vi "Lab Panel V5.28.vi"() -> ()   [LabVIEW 2013] (continued)
              n182 = local write "LAB deg C"(w197) -> ()
              n183 = global write "Global display 4.vi" "LAB deg C"(w197) -> ()
              n184 = local write "OFF amps"(1.5) -> ()
              n185 = local write "ON amps"(20.0) -> ()
              n186 = local write "VOLTS"(250.0) -> ()
              n187 = local write "PF"(0.5) -> ()
            }
            frame #1 {
              n188 = for {
                N: 3 -> [_]
                w243 = TRUE
                n189 = local read "Simulate"() -> (w205:bool)
                n190 = local write "Temp read loop"(0) -> ()
                n191 = case shown="True" w205 {
                  frame False {
                  }
                  frame True {
                    w245 = 20
                    n192 = local write "Ambient Volts"(2.92) -> ()
                    n193 = global write "Global display 3.vi" "Ref deg C"(w245) -> ()
                    n194 = local write "Ref deg C"(w245) -> ()
                  }
                }
                n195 = call "sub vi - GET ALL TEMP v7.vi"("LA01-EN"=w243, "simulate"=w205, "LA02-EN"=w243, "LA03-EN"=w243, "LA04-EN"=w243, "LA05-EN"=w243, "Gen Cal Value"=1) -> ("ID"=w204:T24, "LA01 TEMP"=w241:T25, "LA02 TEMP"=w234:T25, "LA03 TEMP"=w227:T25, "LA04 TEMP"=w220:T25, "LA05 TEMP"=w213:T25)  [unwired: 1 in, 2 out]
                n196 = local write "LAB05 TEMP"(w213) -> ()
                n197 = local write "LAB04 TEMP"(w220) -> ()
                n198 = Unbundle(w227) -> ("T1"=w224:dbl, "T2"=w223:dbl, "T3"=w222:dbl, "T4"=w221:dbl)  [unwired: 2 out]
                n199 = Unbundle(w241) -> ("T1"=w239:dbl, "T2"=w238:dbl, "T3"=w237:dbl, "T4"=w236:dbl)  [unwired: 2 out]
                n200 = Unbundle(w234) -> ("T1"=w231:dbl, "T2"=w230:dbl, "T3"=w229:dbl, "T4"=w228:dbl)  [unwired: 2 out]
                n201 = Unbundle(w220) -> ("T1"=w218:dbl, "T2"=w217:dbl, "T3"=w216:dbl, "T4"=w215:dbl)  [unwired: 2 out]
                n202 = Unbundle(w213) -> ("T1"=w211:dbl, "T2"=w210:dbl, "T3"=w209:dbl, "T4"=w208:dbl)  [unwired: 2 out]
                n203 = local write "LAB01 TEMP"(w241) -> ()
                n204 = local write "LAB02 TEMP"(w234) -> ()
                n205 = local write "LAB03 TEMP"(w227) -> ()
                n206 = Unbundle(w204) -> ("id1"=→"LAB01-TP":bool, "id2"=→"LAB02-TP":bool, "id3"=→"LAB03-TP":bool, "id4"=→"LAB04-TP":bool, "id5"=→"LAB05-TP":bool)
                n207 = local read "TEMP LA05"() -> (w212:T9)
                n208 = local read "TEMP LA04"() -> (w219:T9)
                n209 = local read "TEMP LA02"() -> (w233:T9)
                n210 = local read "TEMP LA03"() -> (w226:T9)
                n211 = local read "TEMP LA01"() -> (w240:T9)
                n212 = Bundle(cluster=w226, "TL-1"=w224, "TN-1"=w223, "TL-2"=w222, "TN-2"=w221) -> (w225:T9)  [unwired: 4 in]
                n213 = Bundle(cluster=w240, "TL-1"=w239, "TN-1"=w238, "TL-2"=w237, "TN-2"=w236) -> (w235:T9)  [unwired: 4 in]
                n214 = Bundle(cluster=w233, "TL-1"=w231, "TN-1"=w230, "TL-2"=w229, "TN-2"=w228) -> (w232:T9)  [unwired: 4 in]
                n215 = Bundle(cluster=w219, "TL-1"=w218, "TN-1"=w217, "TL-2"=w216, "TN-2"=w215) -> (w214:T9)  [unwired: 4 in]
                n216 = Bundle(cluster=w212, "TL-1"=w211, "TN-1"=w210, "TL-2"=w209, "TN-2"=w208) -> (w207:T9)  [unwired: 4 in]
                n217 = local write "TEMP LA03"(w225) -> ()
                n218 = local write "TEMP LA01"(w235) -> ()
                n219 = local write "TEMP LA02"(w232) -> ()
                n220 = local write "TEMP LA05"(w207) -> ()
                n221 = local write "TEMP LA04"(w214) -> ()
              }
            }
            frame #2 {
              w254 = 0
              n222 = local read "LAB01 TEMP"() -> (w256:T12)
              n223 = local read "SIG LAB01-2"() -> (w251:T2)
              n224 = Unbundle By Name(w256) -> ("T1 Live"=w249:dbl, "T1 Neut"=w248:dbl, "T2 Live"=w247:dbl, "T2 Neut"=w246:dbl)  [unwired: 2 out]
              n225 = local read "SIG LAB01-1"() -> (w253:T2)
              n226 = local read "TEMP LA01"() -> (w257:T9)
              n227 = Bundle By Name(cluster=w257, "TL-1"=w249, "TN-1"=w248, "TL-2"=w247, "TN-2"=w246, "TL -1COUNT"=w254, "TN-1 COUNT"=w254, "TL-2 COUNT"=w254, "TN-2 COUNT"=w254) -> (w255:T9)
              n228 = Bundle(cluster=w253, "Tmp Live"=w249, "Tmp Neut"=w248) -> (w252:T2)  [unwired: 3 in]
              n229 = Bundle(cluster=w251, "Tmp Live"=w247, "Tmp Neut"=w246) -> (w250:T2)  [unwired: 3 in]
              n230 = local write "SIG LAB01-2"(w250) -> ()
              n231 = local write "SIG LAB01-1"(w252) -> ()
              n232 = local write "TEMP LA01"(w255) -> ()
            }
            frame #3 {
              w266 = 0
              n233 = local read "LAB02 TEMP"() -> (w268:T12)
              n234 = Unbundle By Name(w268) -> ("T1 Live"=w261:dbl, "T1 Neut"=w260:dbl, "T2 Live"=w259:dbl, "T2 Neut"=w258:dbl)  [unwired: 2 out]
              n235 = local read "SIG LAB02-1"() -> (w265:T2)
              n236 = local read "SIG LAB02-2"() -> (w264:T2)
              n237 = local read "TEMP LA02"() -> (w269:T9)
              n238 = Bundle By Name(cluster=w269, "TL-1"=w261, "TN-1"=w260, "TL-2"=w259, "TN-2"=w258, "TL -1COUNT"=w266, "TN-1 COUNT"=w266, "TL-2 COUNT"=w266, "TN-2 COUNT"=w266) -> (w267:T9)
              n239 = Bundle(cluster=w264, "Tmp Live"=w259, "Tmp Neut"=w258) -> (w262:T2)  [unwired: 3 in]
              n240 = Bundle(cluster=w265, "Tmp Live"=w261, "Tmp Neut"=w260) -> (w263:T2)  [unwired: 3 in]
              n241 = local write "TEMP LA02"(w267) -> ()
              n242 = local write "SIG LAB02-1"(w263) -> ()
              n243 = local write "SIG LAB02-2"(w262) -> ()
            }
            frame #4 {
              w278 = 0
              n244 = local read "LAB03 TEMP"() -> (w280:T12)
              n245 = Unbundle By Name(w280) -> ("T1 Live"=w273:dbl, "T1 Neut"=w272:dbl, "T2 Live"=w271:dbl, "T2 Neut"=w270:dbl)  [unwired: 2 out]
              n246 = local read "SIG LAB03-1"() -> (w277:T2)
              n247 = local read "SIG LAB03-2"() -> (w276:T2)
              n248 = local read "TEMP LA03"() -> (w281:T9)
              n249 = Bundle By Name(cluster=w281, "TL-1"=w273, "TN-1"=w272, "TL-2"=w271, "TN-2"=w270, "TL -1COUNT"=w278, "TN-1 COUNT"=w278, "TL-2 COUNT"=w278, "TN-2 COUNT"=w278) -> (w279:T9)
              n250 = Bundle(cluster=w276, "Tmp Live"=w271, "Tmp Neut"=w270) -> (w274:T2)  [unwired: 3 in]
              n251 = Bundle(cluster=w277, "Tmp Live"=w273, "Tmp Neut"=w272) -> (w275:T2)  [unwired: 3 in]
              n252 = local write "TEMP LA03"(w279) -> ()
              n253 = local write "SIG LAB03-2"(w274) -> ()
              n254 = local write "SIG LAB03-1"(w275) -> ()
            }
            frame #5 {
              w290 = 0
              n255 = local read "LAB04 TEMP"() -> (w292:T12)
              n256 = Unbundle By Name(w292) -> ("T1 Live"=w285:dbl, "T1 Neut"=w284:dbl, "T2 Live"=w283:dbl, "T2 Neut"=w282:dbl)  [unwired: 2 out]
              n257 = local read "SIG LAB04-2"() -> (w288:T2)
              n258 = local read "SIG LAB04-1"() -> (w289:T2)
              n259 = local read "TEMP LA04"() -> (w293:T9)
              n260 = Bundle By Name(cluster=w293, "TL-1"=w285, "TN-1"=w284, "TL-2"=w283, "TN-2"=w282, "TL -1COUNT"=w290, "TN-1 COUNT"=w290, "TL-2 COUNT"=w290, "TN-2 COUNT"=w290) -> (w291:T9)
              n261 = Bundle(cluster=w288, "Tmp Live"=w283, "Tmp Neut"=w282) -> (w286:T2)  [unwired: 3 in]
              n262 = Bundle(cluster=w289, "Tmp Live"=w285, "Tmp Neut"=w284) -> (w287:T2)  [unwired: 3 in]
              n263 = local write "SIG LAB04-2"(w286) -> ()
              n264 = local write "TEMP LA04"(w291) -> ()
              n265 = local write "SIG LAB04-1"(w287) -> ()
            }
            frame #6 {
              w302 = 0
              n266 = local read "LAB05 TEMP"() -> (w304:T12)
              n267 = Unbundle By Name(w304) -> ("T1 Live"=w297:dbl, "T1 Neut"=w296:dbl, "T2 Live"=w295:dbl, "T2 Neut"=w294:dbl)  [unwired: 2 out]
              n268 = local read "SIG LAB05-2"() -> (w300:T2)
              n269 = local read "SIG LAB05-1"() -> (w301:T2)
              n270 = local read "TEMP LA05"() -> (w305:T9)
              n271 = Bundle By Name(cluster=w305, "TL-1"=w297, "TN-1"=w296, "TL-2"=w295, "TN-2"=w294, "TL -1COUNT"=w302, "TN-1 COUNT"=w302, "TL-2 COUNT"=w302, "TN-2 COUNT"=w302) -> (w303:T9)
              n272 = Bundle(cluster=w300, "Tmp Live"=w295, "Tmp Neut"=w294) -> (w298:T2)  [unwired: 3 in]
              n273 = Bundle(cluster=w301, "Tmp Live"=w297, "Tmp Neut"=w296) -> (w299:T2)  [unwired: 3 in]
              n274 = local write "SIG LAB05-2"(w298) -> ()
              n275 = local write "SIG LAB05-1"(w299) -> ()
              n276 = local write "TEMP LA05"(w303) -> ()
            }
          }
        }
        frame #11 {
          # "create analog task"
          n277 = local read "Simulate"() -> (w306:bool)
          n278 = case shown="False" w306 {
            frame False {
              n279 = local read "SAMPLES"() -> (w309:dbl)
              n280 = local read "RATE (Hz)"() -> (w310:dbl)
              n281 = call "sub vi - AI USB4704 (3)  Create Task v4.vi"("Rate Hz"=w310, "Samples"=w309) -> ("TASK USB 0"=→"AI Task0":i32, "TASK USB 1"=→"AI Task1":i32, "TASK USB 2"=→"AI Task2":i32, "AI Task Er"=w307:bool)  [unwired: 9 in, 1 out]
              n282 = local write "Reset Error"(w307) -> ()
              "AI Task" <- TRUE
            }
            frame True {
            }
          }
        }
        frame #12 {
          # "enable front panel, all settings done"
          n283 = property on="Tab Control 2" class="TabCtl (strict)"("DisabledEnum"=T16."Enabled" ("Disabled")) -> ()  [unwired: 2 in, 2 out]
          n284 = property on="Tab Control 2" class="TabCtl (strict)"("Value"=0) -> ()  [unwired: 2 in, 2 out]
        }
        frame #13 {
          n285 = property on="Tab Control 2" class="TabCtl (strict)"("Value"=0) -> ()  [unwired: 2 in, 2 out]
        }
      }
    }
    frame #2 {
      w317 = 250.0
      # "frames that only action on certain cycles, 13, 14, 15, 16, 19, 21"
      n286 = node-c288(w317) -> (w319:T18)  [unwired: 3 in]
      n287 = timed-loop {
        timing: w319 -> [_]
        timing-out: [_] -> w318
        tunnel: w317 -> [w320]
        i -> [w346]
        stop <- w321 stop-if-true
        n288 = node-c288() -> ()  [unwired: 1 in, 1 out]
        n289 = local read "Resets Done"() -> (w325:dbl)
        n290 = local read "SELECT LAB05-2"() -> (w326:T3)
        n291 = local read "SELECT LAB05-1"() -> (w327:T3)
        n292 = local read "SELECT LAB04-2"() -> (w328:T3)
        n293 = local read "SELECT LAB03-1"() -> (w331:T3)
        n294 = local read "SELECT LAB02-2"() -> (w332:T3)
        n295 = local read "SELECT LAB01-1"() -> (w335:T3)
        n296 = local read "SELECT LAB03-2"() -> (w330:T3)
        n297 = local read "SELECT LAB01-2"() -> (w334:T3)
        n298 = local read "SELECT LAB04-1"() -> (w329:T3)
        n299 = Greater?(x=w325, y=50) -> (0:w322:bool)
        n300 = local read "SELECT LAB02-1"() -> (w333:T3)
        n301 = local read "run lab03-2"() -> (w340:bool)
        n302 = local read "run lab04-1"() -> (w339:bool)
        n303 = local read "run lab05-1"() -> (w337:bool)
        n304 = local read "run lab04-2"() -> (w338:bool)
        n305 = local read "run lab05-2"() -> (w336:bool)
        n306 = local read "run lab03-1"() -> (w341:bool)
        n307 = local read "run lab02-2"() -> (w342:bool)
        n308 = local read "run lab02-1"() -> (w343:bool)
        n309 = local read "run lab01-1"() -> (w345:bool)
        n310 = local read "run lab01-2"() -> (w344:bool)
        n311 = Or(x=w322, y="stop") -> (x .or. y?=w321:bool)
        n312 = global write "Global display 1.vi" "stop disp"(w321) -> ()
        n313 = stacked-sequence {
          seq-local: [_ _ w425 _ _ _ _ _ _ _ _ _ _ _ _ _ _ _ _ _ _ _ _ _ _] -> [_ _ _ _ _ _ w2526 _ _ _ _ _ _ _ _ _ _ _ _ _ _ _ _ _ _]
          seq-local: [_ _ w424 _ _ _ _ _ _ _ _ _ _ _ _ _ _ _ _ _ _ _ _ _ _] -> [_ _ _ _ _ _ w2525 _ _ _ _ _ _ _ _ _ _ _ _ _ _ _ _ _ _]
          seq-local: [_ _ w411 _ _ _ _ _ _ _ _ _ _ _ _ _ _ _ _ _ _ _ _ _ _] -> [_ _ _ _ _ _ w2524 _ _ _ _ _ _ _ _ _ _ _ _ _ _ _ _ _ _]
          seq-local: [_ _ w410 _ _ _ _ _ _ _ _ _ _ _ _ _ _ _ _ _ _ _ _ _ _] -> [_ _ _ _ _ _ w2523 _ _ _ _ _ _ _ _ _ _ _ _ _ _ _ _ _ _]
          seq-local: [_ _ w409 _ _ _ _ _ _ _ _ _ _ _ _ _ _ _ _ _ _ _ _ _ _] -> [_ _ _ _ _ _ w2522 _ _ _ _ _ _ _ _ _ _ _ _ _ _ _ _ _ _]
          seq-local: [_ _ w408 _ _ _ _ _ _ _ _ _ _ _ _ _ _ _ _ _ _ _ _ _ _] -> [_ _ _ _ _ _ w2521 _ _ _ _ _ _ _ _ _ _ _ _ _ _ _ _ _ _]
          seq-local: [_ _ w407 _ _ _ _ _ _ _ _ _ _ _ _ _ _ _ _ _ _ _ _ _ _] -> [_ _ _ _ _ _ w2520 _ _ _ _ _ _ _ _ _ _ _ _ _ _ _ _ _ _]
          seq-local: [_ _ w406 _ _ _ _ _ _ _ _ _ _ _ _ _ _ _ _ _ _ _ _ _ _] -> [_ _ _ _ _ _ w2519 _ _ _ _ _ _ _ _ _ _ _ _ _ _ _ _ _ _]
          seq-local: [_ _ w405 _ _ _ _ _ _ _ _ _ _ _ _ _ _ _ _ _ _ _ _ _ _] -> [_ _ _ _ _ _ w2518 _ _ _ _ _ _ _ _ _ _ _ _ _ _ _ _ _ _]
          seq-local: [_ _ w404 _ _ _ _ _ _ _ _ _ _ _ _ _ _ _ _ _ _ _ _ _ _] -> [_ _ _ _ _ _ w2517 _ _ _ _ _ _ _ _ _ _ _ _ _ _ _ _ _ _]
          seq-local: [_ _ _ _ _ _ _ _ _ _ _ _ w3660 _ _ _ _ _ _ _ _ _ _ _ _] -> [_ _ _ _ _ _ _ _ _ _ _ _ _ w3692 _ _ _ _ _ _ _ _ _ _ _]
          tunnel: w345 -> [_ _ _ w441 w689 w2116 w2546 w2862 w3349 _ _ _ _ _ w3976 _ w4933 _ _ w5224 w5528 w5709 _ _ _]
          tunnel: w344 -> [_ _ _ w440 w687 w2115 w2545 w2863 w3348 _ _ _ _ _ w3975 _ w4931 _ _ w5223 w5527 w5707 _ _ _]
          tunnel: w343 -> [_ _ _ w439 w685 w2114 w2544 w2861 w3347 _ _ _ _ _ w3974 _ w4929 _ _ w5222 w5526 w5706 _ _ _]
          tunnel: w342 -> [_ _ _ w438 w683 w2113 w2543 w2860 w3346 _ _ _ _ _ w3973 _ w4927 _ _ w5221 w5525 w5705 _ _ _]
          tunnel: w341 -> [_ _ _ w437 w681 w2112 w2542 w2859 w3345 _ _ _ _ _ w3972 _ w4925 _ _ w5220 w5524 w5704 _ _ _]
          tunnel: w340 -> [_ _ _ w436 w679 w2111 w2541 w2858 w3344 _ _ _ _ _ w3971 _ w4923 _ _ w5219 w5523 w5703 _ _ _]
          tunnel: w339 -> [_ _ _ w435 w677 w2110 w2540 w2857 w3343 _ _ _ _ _ w3970 _ w4921 _ _ w5218 w5522 w5702 _ _ _]
          tunnel: w338 -> [_ _ _ w434 w675 w2109 w2539 w2856 w3342 _ _ _ _ _ w3969 _ w4919 _ _ w5217 w5521 w5701 _ _ _]
          tunnel: w337 -> [_ _ _ w433 w673 w2108 w2538 w2855 w3341 _ _ _ _ _ w3968 _ w4917 _ _ w5216 w5520 w5700 _ _ _]
          tunnel: w336 -> [_ _ _ w432 w671 w2107 w2537 w2854 w3340 _ _ _ _ _ w3967 _ w4915 _ _ w5215 w5519 w5699 _ _ _]
          tunnel: w335 -> [_ _ _ _ w688 w2106 w2536 _ _ _ _ _ _ _ _ _ w4935 _ _ _ _ _ w6165 _ _]
          tunnel: w334 -> [_ _ _ _ w686 w2105 w2535 _ _ _ _ _ _ _ _ _ w4930 _ _ _ _ _ w6164 _ _]
          tunnel: w333 -> [_ _ _ _ w684 w2104 w2534 _ _ _ _ _ _ _ _ _ w4928 _ _ _ _ _ w6163 _ _]
          tunnel: w332 -> [_ _ _ _ w682 w2103 w2533 _ _ _ _ _ _ _ _ _ w4926 _ _ _ _ _ w6162 _ _]
          tunnel: w331 -> [_ _ _ _ w680 w2102 w2532 _ _ _ _ _ _ _ _ _ w4924 _ _ _ _ _ w6161 _ _]
          tunnel: w330 -> [_ _ _ _ w678 w2101 w2531 _ _ _ _ _ _ _ _ _ w4922 _ _ _ _ _ w6160 _ _]
          tunnel: w329 -> [_ _ _ _ w676 w2100 w2530 _ _ _ _ _ _ _ _ _ w4920 _ _ _ _ _ w6159 _ _]
          tunnel: w328 -> [_ _ _ _ w674 w2099 w2529 _ _ _ _ _ _ _ _ _ w4918 _ _ _ _ _ w6158 _ _]
          tunnel: w327 -> [_ _ _ _ w672 w2098 w2528 _ _ _ _ _ _ _ _ _ w4916 _ _ _ _ _ w6157 _ _]
          tunnel: w326 -> [_ _ _ _ w670 w2097 w2527 _ _ _ _ _ _ _ _ _ w4914 _ _ _ _ _ w6156 _ _]
          tunnel: w322 -> [_ _ _ _ _ _ _ _ _ _ _ _ _ _ _ _ _ _ _ _ _ _ _ _ w6268]
          tunnel: w321 -> [_ _ _ _ _ _ _ _ _ _ _ _ _ _ _ _ _ _ _ _ _ _ _ _ w6267]
          tunnel: w320 -> [_ w361 _ _ _ _ _ _ _ _ _ _ _ _ _ _ _ _ _ _ _ _ _ _ _]
          frame #0 {
            n314 = local read "AI Task"() -> (w349:bool)
            n315 = global write "Global 1.vi" "RATE(Hz)"("RATE (Hz)") -> ()
            n316 = case shown="True" w349 {
              frame False {
              }
              frame True {
                n317 = local read "SAMPLES"() -> (w351:dbl)
                n318 = local read "AI Task2"() -> (w357:dbl)
                n319 = local read "AI Task1"() -> (w358:dbl)
                n320 = local read "AI Task0"() -> (w359:dbl)
                n321 = call "sub vi - AI USB4704 (3) v73.vi"("Task0"=w359, "Task1"=w358, "Task2"=w357, "SAMPLES"=w351) -> ("data 0"=→"AI data 0" →"AI Data 0":waveform(dbl)[], "data 1"=→"AI data 1" →"AI Data 1":waveform(dbl)[], "data 2"=→"AI data 2" →"AI Data 2":waveform(dbl)[], "loop time"=→"AI loop time":dbl, "error array"=→"AI Error":errorcluster[])  [unwired: 7 in]
              }
            }
          }
          frame #1 {
            w368 = FALSE
            # "set up cycle control"
            n322 = local read "jig cycle"() -> (w372:dbl)
            n323 = local read "Amps Fail level"() -> (w366:dbl)
            n324 = local read "Simulate"() -> (w363:bool)
            n325 = Divide(x=w361, y=1000.0) -> (x/y=w360:dbl)
            n326 = Divide(x="JIG ON TIME (S)", y=w360) -> (x/y=→"on loops":dbl)
            n327 = Divide(x="JIG OFF TIME (S)", y=w360) -> (x/y=→"off loops":dbl)
            n328 = Increment(x=w372) -> (x+1=w371:dbl)
            n329 = local write "Simulate IND"(w363) -> ()
            n330 = global write "Global display 3.vi" "Amps Fail"(w366) -> ()
            n331 = local write "TEMP"(w368) -> ()
            n332 = local write "AI"(w368) -> ()
            n333 = local read "Network Directory"() -> (w365:path)
            n334 = local write "jig cycle"(w371) -> ()
            n335 = call "sub vi - check network dir v2.vi"("PATH"=w365) -> ("error"=w364:bool)  [unwired: 10 in]
            n336 = local write "network error"(w364) -> ()
            n337 = global write "Global display 3.vi" "network drive"(w364) -> ()
            n338 = event shown="[1] \"ADMIN\": Value Change" {
              selector: _ -> [_ _]
              dyn-events: _ -> [_ _]
              timeout: 10 -> [_ _]
              event Timeout {
                n339 = event-data() -> ()  [unwired: 1 in, 3 out]
              }
              event "ADMIN": Value Change {
                n340 = event-data() -> ()  [unwired: 1 in, 6 out]
                n341 = stacked-sequence {
                  seq-local: [_ w376 _] -> [_ _ w377]
                  frame #0 {
                    n342 = global write "Global 1.vi" "password"("9949") -> ()
                  }
                  frame #1 {
                    n343 = call "sub vi - password 1.vi"() -> ("RESULT"=w376:bool)  [unwired: 11 in]
                  }
                  frame #2 {
                    w379 = FALSE
                    n344 = property on="Tab Control 2" class="TabCtl (strict)"() -> ("Pages"=w383:refnum<vi>[])  [unwired: 2 in, 2 out]
                    n345 = Select(t=TRUE, s=w377, f=w379) -> (s? t:f=w378:bool)
                    n346 = Index Array(array=w383, index=8) -> (element=w381:refnum<vi>)
                    n347 = property class="Page"(reference=w381, "PageVis"=w378) -> ()  [unwired: 1 in, 2 out]
                    n348 = local write "ADMIN"(w379) -> ()
                  }
                }
              }
            }
          }
          frame #2 {
            w421 = 60.0
            # "convert temperature rise minutes to cycles"
            n349 = local read "SET LAB05-2"() -> (w385:T5)
            n350 = local read "SET LAB05-1"() -> (w387:T5)
            n351 = local read "SET LAB04-2"() -> (w389:T5)
            n352 = local read "SET LAB01-1"() -> (w403:T5)
            n353 = local read "SET LAB01-2"() -> (w401:T5)
            n354 = local read "SET LAB02-2"() -> (w397:T5)
            n355 = local read "SET LAB04-1"() -> (w391:T5)
            n356 = local read "SET LAB03-1"() -> (w395:T5)
            n357 = local read "SET LAB03-2"() -> (w393:T5)
            n358 = local read "SET LAB02-1"() -> (w399:T5)
            n359 = local read "JIG OFF TIME (S)"() -> (w426:dbl)
            n360 = local read "JIG ON TIME (S)"() -> (w427:dbl)
            n361 = Unbundle(w385) -> ("T-RISE mins"=w384:dbl)  [unwired: 4 out]
            n362 = Unbundle(w387) -> ("T-RISE mins"=w386:dbl)  [unwired: 4 out]
            n363 = Unbundle(w403) -> ("T-RISE mins"=w402:dbl)  [unwired: 4 out]
            n364 = Unbundle(w389) -> ("T-RISE mins"=w388:dbl)  [unwired: 4 out]
            n365 = Unbundle(w401) -> ("T-RISE mins"=w400:dbl)  [unwired: 4 out]
            n366 = Unbundle(w399) -> ("T-RISE mins"=w398:dbl)  [unwired: 4 out]
            n367 = Unbundle(w391) -> ("T-RISE mins"=w390:dbl)  [unwired: 4 out]
            n368 = Unbundle(w397) -> ("T-RISE mins"=w396:dbl)  [unwired: 4 out]
            n369 = Unbundle(w393) -> ("T-RISE mins"=w392:dbl)  [unwired: 4 out]
            n370 = Unbundle(w395) -> ("T-RISE mins"=w394:dbl)  [unwired: 4 out]
            n371 = Add(x=w427, y=w426) -> (x+y=w420:dbl)
            n372 = Multiply(x=w421, y=w392) -> (x*y=w416:dbl)
            n373 = Multiply(x=w421, y=w390) -> (x*y=w415:dbl)
            n374 = Multiply(x=w421, y=w388) -> (x*y=w414:dbl)
            n375 = Multiply(x=w421, y=w386) -> (x*y=w413:dbl)
            n376 = Multiply(x=w421, y=w384) -> (x*y=w412:dbl)
            n377 = Multiply(x=w421, y=w400) -> (x*y=w422:dbl)
            n378 = Multiply(x=w421, y=w394) -> (x*y=w417:dbl)
            n379 = Multiply(x=w421, y=w402) -> (x*y=w423:dbl)
            n380 = Multiply(x=w421, y=w398) -> (x*y=w419:dbl)
            n381 = Multiply(x=w421, y=w396) -> (x*y=w418:dbl)
            n382 = Divide(x=w413, y=w420) -> (x/y=w405:dbl)
            n383 = Divide(x=w414, y=w420) -> (x/y=w406:dbl)
            n384 = Divide(x=w415, y=w420) -> (x/y=w407:dbl)
            n385 = Divide(x=w412, y=w420) -> (x/y=w404:dbl)
            n386 = Divide(x=w417, y=w420) -> (x/y=w409:dbl)
            n387 = Divide(x=w423, y=w420) -> (x/y=w425:dbl)
            n388 = Divide(x=w422, y=w420) -> (x/y=w424:dbl)
            n389 = Divide(x=w419, y=w420) -> (x/y=w411:dbl)
            n390 = Divide(x=w418, y=w420) -> (x/y=w410:dbl)
            n391 = Divide(x=w416, y=w420) -> (x/y=w408:dbl)
          }
          frame #3 {
            # "control cycle loops"
            n392 = local read "JIG OFF TIME (S)"() -> (w430:dbl)
            n393 = local read "JIG ON TIME (S)"() -> (w429:dbl)
            n394 = local read "jig cycle"() -> (w443:dbl)
            n395 = local read "on loops"() -> (w445:dbl)
            n396 = local read "off loops"() -> (w444:dbl)
            n397 = Add(x=w430, y=w429) -> (x+y=w428:dbl)
            n398 = Add(x=w445, y=w444) -> (x+y=w431:dbl)
            n399 = Greater Or Equal?(x=w443, y=w431) -> (x >= y?=w442:bool)
            n400 = case shown="True" w442 {
              tunnel: w441 -> [_ w479]
              tunnel: w440 -> [_ w478]
              tunnel: w439 -> [_ w477]
              tunnel: w438 -> [_ w476]
              tunnel: w437 -> [_ w475]
              tunnel: w436 -> [_ w474]
              tunnel: w435 -> [_ w473]
              tunnel: w434 -> [_ w472]
              tunnel: w433 -> [_ w471]
              tunnel: w432 -> [_ w470]
              tunnel: w428 -> [_ w469]
              frame False {
              }
              frame True {
                # "increment cycle value and convert cycles to minutes for temp rise"
                n401 = stacked-sequence {
                  frame #0 {
                    n402 = local read "Temp read loop"() -> (w482:dbl)
                    n403 = Increment(x=w482) -> (x+1=w481:dbl)
                    n404 = local write "Temp read loop"(w481) -> ()
                  }
                  frame #1 {
                    n405 = local read "Temp read loop"() -> (w483:dbl)
                    n406 = Greater?(x=w483, y=20) -> (0:w485:bool)
                    n407 = case shown="True" w485 {
                      frame False {
                      }
                      frame True {
                        n408 = local write "Temp read loop"(1) -> ()
                      }
                    }
                  }
                }
                n409 = local read "JIG RELAY CYCLES"() -> (w468:T8)
                n410 = local read "Temp read loop"() -> (→"Tp Up":dbl)
                n411 = Unbundle By Name(w468) -> ("LAB01-1"=w466:dbl, "LAB01-2"=w464:dbl, "LAB02-1"=w462:dbl, "LAB02-2"=w460:dbl, "LAB03-1"=w458:dbl, "LAB03-2"=w456:dbl, "LAB04-1"=w454:dbl, "LAB04-2"=w452:dbl, "LAB05-1"=w450:dbl, "LAB05-2"=w448:dbl)
                n412 = stacked-sequence {
                  tunnel: w479 -> [w497 _ _ _ _ _ _ _ _ _]
                  tunnel: w478 -> [_ w514 _ _ _ _ _ _ _ _]
                  tunnel: w477 -> [_ _ w531 _ _ _ _ _ _ _]
                  tunnel: w476 -> [_ _ _ w548 _ _ _ _ _ _]
                  tunnel: w475 -> [_ _ _ _ w565 _ _ _ _ _]
                  tunnel: w474 -> [_ _ _ _ _ w582 _ _ _ _]
                  tunnel: w473 -> [_ _ _ _ _ _ w599 _ _ _]
                  tunnel: w472 -> [_ _ _ _ _ _ _ w616 _ _]
                  tunnel: w471 -> [_ _ _ _ _ _ _ _ w633 _]
                  tunnel: w470 -> [_ _ _ _ _ _ _ _ _ w650]
                  tunnel: w469 -> [w494 w511 w528 w545 w562 w579 w596 w613 w630 w647]
                  tunnel: w466 -> [w488 _ _ _ _ _ _ _ _ _]
                  tunnel: [w487 _ _ _ _ _ _ _ _ _] -> w465
                  tunnel: w464 -> [_ w505 _ _ _ _ _ _ _ _]
                  tunnel: [_ w504 _ _ _ _ _ _ _ _] -> w463
                  tunnel: w462 -> [_ _ w522 _ _ _ _ _ _ _]
                  tunnel: [_ _ w521 _ _ _ _ _ _ _] -> w461
                  tunnel: w460 -> [_ _ _ w539 _ _ _ _ _ _]
                  tunnel: [_ _ _ w538 _ _ _ _ _ _] -> w459
                  tunnel: w458 -> [_ _ _ _ w556 _ _ _ _ _]
                  tunnel: [_ _ _ _ w555 _ _ _ _ _] -> w457
                  tunnel: w456 -> [_ _ _ _ _ w573 _ _ _ _]
                  tunnel: [_ _ _ _ _ w572 _ _ _ _] -> w455
                  tunnel: w454 -> [_ _ _ _ _ _ w590 _ _ _]
                  tunnel: [_ _ _ _ _ _ w589 _ _ _] -> w453
                  tunnel: w452 -> [_ _ _ _ _ _ _ w607 _ _]
                  tunnel: [_ _ _ _ _ _ _ w606 _ _] -> w451
                  tunnel: w450 -> [_ _ _ _ _ _ _ _ w624 _]
                  tunnel: [_ _ _ _ _ _ _ _ w623 _] -> w449
                  tunnel: w448 -> [_ _ _ _ _ _ _ _ _ w641]
                  tunnel: [_ _ _ _ _ _ _ _ _ w640] -> w447
                  frame #0 {
                    n413 = local read "DISP LAB01-1"() -> (w492:T4)
                    n414 = Unbundle(w492) -> ("CYCLE"=w493:dbl)  [unwired: 2 out]
                    n415 = case shown="True" w497 {
                      tunnel: w493 -> [w499 w503]
                      tunnel: [w499 w502] -> w491
                      tunnel: w488 -> [w498 w501]
                      tunnel: [w498 w500] -> w487
                      frame False {
                      }
                      frame True {
                        n416 = Increment(x=w501) -> (x+1=w500:dbl)
                        n417 = Increment(x=w503) -> (x+1=w502:dbl)
                      }
                    }
                    n418 = Multiply(x=w491, y=w494) -> (x*y=w495:dbl)
                    n419 = Divide(x=w495, y=60.0) -> (x/y=w490:dbl)
                    n420 = Bundle(cluster=w492, "CYCLE"=w491, "MINS"=w490) -> (w489:T4)  [unwired: 1 in]
                    n421 = local write "DISP LAB01-1"(w489) -> ()
                  }
                  frame #1 {
                    n422 = local read "DISP LAB01-2"() -> (w509:T4)
                    n423 = Unbundle(w509) -> ("CYCLE"=w510:dbl)  [unwired: 2 out]
                    n424 = case shown="True" w514 {
                      tunnel: w510 -> [w516 w520]
                      tunnel: [w516 w519] -> w507
                      tunnel: w505 -> [w515 w518]
                      tunnel: [w515 w517] -> w504
                      frame False {
                      }
                      frame True {
                        n425 = Increment(x=w518) -> (x+1=w517:dbl)
                        n426 = Increment(x=w520) -> (x+1=w519:dbl)
                      }
                    }
                    n427 = Multiply(x=w507, y=w511) -> (x*y=w512:dbl)
                    n428 = Divide(x=w512, y=60.0) -> (x/y=w506:dbl)
                    n429 = Bundle(cluster=w509, "CYCLE"=w507, "MINS"=w506) -> (w508:T4)  [unwired: 1 in]
                    n430 = local write "DISP LAB01-2"(w508) -> ()
                  }
                  frame #2 {
                    n431 = local read "DISP LAB02-1"() -> (w526:T4)
                    n432 = Unbundle(w526) -> ("CYCLE"=w527:dbl)  [unwired: 2 out]
                    n433 = case shown="True" w531 {
                      tunnel: [w533 w537] -> w524
                      tunnel: w527 -> [w533 w536]
                      tunnel: w522 -> [w532 w535]
                      tunnel: [w532 w534] -> w521
                      frame False {
                      }
                      frame True {
                        n434 = Increment(x=w535) -> (x+1=w534:dbl)
                        n435 = Increment(x=w536) -> (x+1=w537:dbl)
                      }
                    }
                    n436 = Multiply(x=w524, y=w528) -> (x*y=w529:dbl)
                    n437 = Divide(x=w529, y=60.0) -> (x/y=w523:dbl)
                    n438 = Bundle(cluster=w526, "CYCLE"=w524, "MINS"=w523) -> (w525:T4)  [unwired: 1 in]
                    n439 = local write "DISP LAB02-1"(w525) -> ()
                  }
                  frame #3 {
                    n440 = local read "DISP LAB02-2"() -> (w543:T4)
                    n441 = Unbundle(w543) -> ("CYCLE"=w544:dbl)  [unwired: 2 out]
                    n442 = case shown="True" w548 {
                      tunnel: [w550 w554] -> w542
                      tunnel: w544 -> [w550 w553]
                      tunnel: w539 -> [w549 w552]
                      tunnel: [w549 w551] -> w538
                      frame False {
                      }
                      frame True {
                        n443 = Increment(x=w552) -> (x+1=w551:dbl)
                        n444 = Increment(x=w553) -> (x+1=w554:dbl)
                      }
                    }
                    n445 = Multiply(x=w542, y=w545) -> (x*y=w546:dbl)
                    n446 = Divide(x=w546, y=60.0) -> (x/y=w541:dbl)
                    n447 = Bundle(cluster=w543, "CYCLE"=w542, "MINS"=w541) -> (w540:T4)  [unwired: 1 in]
                    n448 = local write "DISP LAB02-2"(w540) -> ()
                  }
                  frame #4 {
                    n449 = local read "DISP LAB03-1"() -> (w560:T4)
                    n450 = Unbundle(w560) -> ("CYCLE"=w561:dbl)  [unwired: 2 out]
                    n451 = case shown="True" w565 {
                      tunnel: [w567 w571] -> w557
                      tunnel: w561 -> [w567 w570]
                      tunnel: w556 -> [w566 w569]
                      tunnel: [w566 w568] -> w555
                      frame False {
                      }
                      frame True {
                        n452 = Increment(x=w569) -> (x+1=w568:dbl)
                        n453 = Increment(x=w570) -> (x+1=w571:dbl)
                      }
                    }
                    n454 = Multiply(x=w557, y=w562) -> (x*y=w563:dbl)
                    n455 = Divide(x=w563, y=60.0) -> (x/y=w558:dbl)
                    n456 = Bundle(cluster=w560, "CYCLE"=w557, "MINS"=w558) -> (w559:T4)  [unwired: 1 in]
                    n457 = local write "DISP LAB03-1"(w559) -> ()
                  }
                  frame #5 {
                    n458 = local read "DISP LAB03-2"() -> (w577:T4)
                    n459 = Unbundle(w577) -> ("CYCLE"=w578:dbl)  [unwired: 2 out]
                    n460 = case shown="True" w582 {
                      tunnel: [w584 w588] -> w576
                      tunnel: w578 -> [w584 w587]
                      tunnel: w573 -> [w583 w586]
                      tunnel: [w583 w585] -> w572
                      frame False {
                      }
                      frame True {
                        n461 = Increment(x=w586) -> (x+1=w585:dbl)
                        n462 = Increment(x=w587) -> (x+1=w588:dbl)
                      }
                    }
                    n463 = Multiply(x=w576, y=w579) -> (x*y=w580:dbl)
                    n464 = Divide(x=w580, y=60.0) -> (x/y=w575:dbl)
                    n465 = Bundle(cluster=w577, "CYCLE"=w576, "MINS"=w575) -> (w574:T4)  [unwired: 1 in]
                    n466 = local write "DISP LAB03-2"(w574) -> ()
                  }
                  frame #6 {
                    n467 = local read "DISP LAB04-1"() -> (w594:T4)
                    n468 = Unbundle(w594) -> ("CYCLE"=w595:dbl)  [unwired: 2 out]
                    n469 = case shown="True" w599 {
                      tunnel: [w601 w605] -> w592
                      tunnel: w595 -> [w601 w604]
                      tunnel: w590 -> [w600 w603]
                      tunnel: [w600 w602] -> w589
                      frame False {
                      }
                      frame True {
                        n470 = Increment(x=w603) -> (x+1=w602:dbl)
                        n471 = Increment(x=w604) -> (x+1=w605:dbl)
                      }
                    }
                    n472 = Multiply(x=w592, y=w596) -> (x*y=w597:dbl)
                    n473 = Divide(x=w597, y=60.0) -> (x/y=w591:dbl)
                    n474 = Bundle(cluster=w594, "CYCLE"=w592, "MINS"=w591) -> (w593:T4)  [unwired: 1 in]
                    n475 = local write "DISP LAB04-1"(w593) -> ()
                  }
                  frame #7 {
                    n476 = local read "DISP LAB04-2"() -> (w611:T4)
                    n477 = Unbundle(w611) -> ("CYCLE"=w612:dbl)  [unwired: 2 out]
                    n478 = case shown="True" w616 {
                      tunnel: [w618 w622] -> w609
                      tunnel: w612 -> [w618 w621]
                      tunnel: w607 -> [w617 w620]
                      tunnel: [w617 w619] -> w606
                      frame False {
                      }
                      frame True {
                        n479 = Increment(x=w620) -> (x+1=w619:dbl)
                        n480 = Increment(x=w621) -> (x+1=w622:dbl)
                      }
                    }
                    n481 = Multiply(x=w609, y=w613) -> (x*y=w615:dbl)
                    n482 = Divide(x=w615, y=60.0) -> (x/y=w608:dbl)
                    n483 = Bundle(cluster=w611, "CYCLE"=w609, "MINS"=w608) -> (w610:T4)  [unwired: 1 in]
                    n484 = local write "DISP LAB04-2"(w610) -> ()
                  }
                  frame #8 {
                    n485 = local read "DISP LAB05-1"() -> (w628:T4)
                    n486 = Unbundle(w628) -> ("CYCLE"=w629:dbl)  [unwired: 2 out]
                    n487 = case shown="True" w633 {
                      tunnel: [w635 w639] -> w626
                      tunnel: w629 -> [w635 w638]
                      tunnel: w624 -> [w634 w637]
                      tunnel: [w634 w636] -> w623
                      frame False {
                      }
                      frame True {
                        n488 = Increment(x=w637) -> (x+1=w636:dbl)
                        n489 = Increment(x=w638) -> (x+1=w639:dbl)
                      }
                    }
                    n490 = Multiply(x=w626, y=w630) -> (x*y=w631:dbl)
                    n491 = Divide(x=w631, y=60.0) -> (x/y=w625:dbl)
                    n492 = Bundle(cluster=w628, "CYCLE"=w626, "MINS"=w625) -> (w627:T4)  [unwired: 1 in]
                    n493 = local write "DISP LAB05-1"(w627) -> ()
                  }
                  frame #9 {
                    n494 = local read "DISP LAB05-2"() -> (w646:T4)
                    n495 = Unbundle(w646) -> ("CYCLE"=w645:dbl)  [unwired: 2 out]
                    n496 = case shown="True" w650 {
                      tunnel: [w652 w656] -> w644
                      tunnel: w645 -> [w652 w655]
                      tunnel: w641 -> [w651 w654]
                      tunnel: [w651 w653] -> w640
                      frame False {
                      }
                      frame True {
                        n497 = Increment(x=w654) -> (x+1=w653:dbl)
                        n498 = Increment(x=w655) -> (x+1=w656:dbl)
                      }
                    }
                    n499 = Multiply(x=w644, y=w647) -> (x*y=w648:dbl)
                    n500 = Divide(x=w648, y=60.0) -> (x/y=w643:dbl)
                    n501 = Bundle(cluster=w646, "CYCLE"=w644, "MINS"=w643) -> (w642:T4)  [unwired: 1 in]
                    n502 = local write "DISP LAB05-2"(w642) -> ()
                  }
                }
                n503 = local write "jig cycle"(0) -> ()
                n504 = Bundle By Name(cluster=w468, "LAB01-1"=w465, "LAB01-2"=w463, "LAB02-1"=w461, "LAB02-2"=w459, "LAB03-1"=w457, "LAB03-2"=w455, "LAB04-1"=w453, "LAB04-2"=w451, "LAB05-1"=w449, "LAB05-2"=w447) -> (w467:T8)
                n505 = local write "JIG RELAY CYCLES"(w467) -> ()
              }
            }
          }
          frame #4 {
            # "START & STOP test RUN switch change, start test if true and stop test if false"
            n506 = Get Date/Time In Seconds() -> (seconds since 1Jan1904=w668:timestamp)
            n507 = local read "C drive data root dir"() -> (w661:path)
            n508 = Format Date/Time String(time format string (%c)="%b\\%a%d", seconds (now)=w668) -> (date/time string=w692:string)  [unwired: 1 in]
            n509 = Format Date/Time String(time format string (%c)="%H%M", seconds (now)=w668) -> (date/time string=w690:string)  [unwired: 1 in]
            n510 = Format Date/Time String(time format string (%c)="LabPanel%Y", seconds (now)=w668) -> (date/time string=w667:string)  [unwired: 1 in]
            n511 = Path To String(path=w661) -> (string=w664:string)
            n512 = global write "Global 1.vi" "C drive root path"(w661) -> ()
            n513 = local read "Ref deg C"() -> (w657:dbl)
            n514 = Concatenate Strings(w664, "\\") -> (w662:string)
            n515 = event shown="[1] \"RUN LAB01-1\": Value Change" {
              selector: _ -> [_ _ _ _ _ _ _ _ _ _ _]
              dyn-events: _ -> [_ _ _ _ _ _ _ _ _ _ _]
              timeout: 10 -> [_ _ _ _ _ _ _ _ _ _ _]
              tunnel: w662 -> [_ w705 w845 w986 w1126 w1266 w1406 w1546 w1686 w1826 w1967]
              tunnel: w692 -> [_ w704 w844 w985 w1125 w1265 w1405 w1545 w1685 w1825 w1966]
              tunnel: w690 -> [_ w702 w843 w984 w1124 w1264 w1404 w1544 w1684 w1824 w1965]
              tunnel: w688 -> [_ w703 _ _ _ _ _ _ _ _ _]
              tunnel: w689 -> [_ _ _ _ _ _ _ _ _ _ _]
              tunnel: w687 -> [_ _ _ _ _ _ _ _ _ _ _]
              tunnel: w686 -> [_ _ w842 _ _ _ _ _ _ _ _]
              tunnel: w685 -> [_ _ _ _ _ _ _ _ _ _ _]
              tunnel: w684 -> [_ _ _ w983 _ _ _ _ _ _ _]
              tunnel: w683 -> [_ _ _ _ _ _ _ _ _ _ _]
              tunnel: w682 -> [_ _ _ _ w1123 _ _ _ _ _ _]
              tunnel: w681 -> [_ _ _ _ _ _ _ _ _ _ _]
              tunnel: w680 -> [_ _ _ _ _ w1263 _ _ _ _ _]
              tunnel: w679 -> [_ _ _ _ _ _ _ _ _ _ _]
              tunnel: w678 -> [_ _ _ _ _ _ w1403 _ _ _ _]
              tunnel: w677 -> [_ _ _ _ _ _ _ _ _ _ _]
              tunnel: w676 -> [_ _ _ _ _ _ _ w1543 _ _ _]
              tunnel: w675 -> [_ _ _ _ _ _ _ _ _ _ _]
              tunnel: w674 -> [_ _ _ _ _ _ _ _ w1683 _ _]
              tunnel: w673 -> [_ _ _ _ _ _ _ _ _ _ _]
              tunnel: w672 -> [_ _ _ _ _ _ _ _ _ w1823 _]
              tunnel: w671 -> [_ _ _ _ _ _ _ _ _ _ _]
              tunnel: w670 -> [_ _ _ _ _ _ _ _ _ _ w1964]
              tunnel: w667 -> [_ w701 w841 w982 w1122 w1262 w1402 w1542 w1682 w1822 w1963]
              tunnel: [_ w700 w840 w981 w1121 w1261 w1401 w1541 w1681 w1821 w1962] -> w665
              tunnel: "RESET CYCLES TO ZERO?" -> [_ w699 w838 w979 w1119 w1259 w1399 w1539 w1679 w1819 w1960]
              tunnel: "YES" -> [_ w698 w837 w978 w1118 w1258 w1398 w1538 w1678 w1818 w1959]
              tunnel: "NO" -> [_ w697 w836 w977 w1117 w1257 w1397 w1537 w1677 w1817 w1958]
              tunnel: w657 -> [_ w694 w835 w975 w1116 w1256 w1396 w1536 w1676 w1816 w1956]
              event Timeout {
                n516 = event-data() -> ()  [unwired: 1 in, 3 out]
              }
              event "RUN LAB01-1": Value Change {
                n517 = event-data() -> ("NewVal"=w695:bool)  [unwired: 1 in, 5 out]
                n518 = local read "SIG LAB01-1"() -> (w696:T2)
                n519 = local write "run lab01-1"(w695) -> ()
                n520 = case shown="False" w695 {
                  tunnel: w705 -> [_ w743]
                  tunnel: w704 -> [_ w742]
                  tunnel: w703 -> [w707 w741]
                  tunnel: w702 -> [_ w740]
                  tunnel: w701 -> [_ w739]
                  tunnel: [w706 w738] -> w700
                  tunnel: w699 -> [_ w737]
                  tunnel: w698 -> [_ w736]
                  tunnel: w697 -> [_ w735]
                  tunnel: w696 -> [_ w734]
                  tunnel: w694 -> [_ w733]
                  frame False {
                    # "stop test"
                    n521 = stacked-sequence {
                      tunnel: w707 -> [_ w719 _]
                      tunnel: [_ w711 _] -> w706
                      frame #0 {
                        n522 = local read "DISP LAB01-1"() -> (w710:T4)
                        n523 = Bundle(cluster=w710, "STATUS"="STOP") -> (w708:T4)  [unwired: 2 in]
                        n524 = local write "DISP LAB01-1"(w708) -> ()
                      }
                      frame #1 {
                        n525 = local read "DISP LAB01-1"() -> (w718:T4)
                        n526 = Unbundle(w718) -> ("CYCLE"=w716:dbl, "MINS"=w717:dbl)  [unwired: 1 out]
                        n527 = case shown="\"CYCLE TEST\"" w719 {
                          tunnel: w717 -> [_ _ w726]
                          tunnel: w716 -> [w724 w725 _]
                          tunnel: [w724 w725 w726] -> w715
                          frame "CHART TEST", Default {
                          }
                          frame "CYCLE TEST" {
                          }
                          frame "T-RISE TEST" {
                          }
                        }
                        n528 = local read "TDMS LAB01-1"() -> (w723:refnum<k34>)
                        n529 = Build Array("STOPPED") -> (w720:string[])
                        n530 = Build Array(w715) -> (w714:dbl[])
                        n531 = TDMS Write(0:w723, 5:"TEST RESULT", 7:w720, 9:w714) -> (4:w712:refnum<k34>, 15:w713:errorcluster)  [unwired: 2 in, 2 out]
                        n532 = TDMS Close(8:w713, 11:w712) -> (0:w711:errorcluster)  [unwired: 1 out]
                      }
                      frame #2 {
                        n533 = stacked-sequence {
                          tunnel: "LAB01-1" -> [w729 w731]
                          frame #0 {
                            n534 = call "sub vi - defrag tdms v1.vi"("panel id"=w729) -> ("error out"=w728:errorcluster)  [unwired: 10 in]
                            n535 = local write "data file error"(w728) -> ()
                          }
                          frame #1 {
                            n536 = call "Save data file (stop) v3.vi"("panel id"=w731) -> ("network file save error"=w730:errorcluster)  [unwired: 9 in, 1 out]
                            n537 = local write "RESULT LAB01-1"(FALSE) -> ()
                            n538 = local write "data file error"(w730) -> ()
                          }
                        }
                      }
                    }
                  }
                  frame True {
                    n539 = stacked-sequence {
                      seq-local: [w745 _] -> [_ w749]
                      tunnel: w743 -> [_ w759]
                      tunnel: w742 -> [_ w758]
                      tunnel: w741 -> [_ w757]
                      tunnel: w740 -> [_ w756]
                      tunnel: w739 -> [_ w755]
                      tunnel: [_ w754] -> w738
                      tunnel: w737 -> [_ w753]
                      tunnel: w736 -> [_ w752]
                      tunnel: w735 -> [_ w751]
                      tunnel: w734 -> [w747 w750]
                      tunnel: w733 -> [_ w748]
                      frame #0 {
                        n540 = Unbundle(w747) -> ("AMPS"=w746:dbl)  [unwired: 4 out]
                        n541 = call "Check For Amps on v1.vi"("ID"="LAB01-1", "amps"=w746) -> ("amps"=w745:bool)  [unwired: 9 in]
                      }
                      frame #1 {
                        n542 = case shown="True" w749 {
                          tunnel: w759 -> [_ w772]
                          tunnel: w758 -> [_ w771]
                          tunnel: w757 -> [_ w770]
                          tunnel: w756 -> [_ w769]
                          tunnel: w755 -> [_ w768]
                          tunnel: [errorcluster {"status"=FALSE, "code"=0, "source"=""} ("error out") w767] -> w754
                          tunnel: w753 -> [_ w766]
                          tunnel: w752 -> [_ w765]
                          tunnel: w751 -> [_ w764]
                          tunnel: w750 -> [_ w763]
                          tunnel: w748 -> [_ w762]
                          frame False {
                            w760 = FALSE
                            n543 = local write "RUN LAB01-1"(w760) -> ()
                            n544 = local write "run lab01-1"(w760) -> ()
                          }
                          frame True {
                            n545 = stacked-sequence {
                              seq-local: [w773 _ _ _ _] -> [_ w794 _ _ _]
                              tunnel: w772 -> [w778 _ _ _ _]
                              tunnel: w771 -> [w774 _ _ _ _]
                              tunnel: w770 -> [w788 _ _ _ _]
                              tunnel: w769 -> [w781 _ _ _ _]
                              tunnel: w768 -> [w776 _ _ _ _]
                              tunnel: [_ w795 _ _ _] -> w767
                              tunnel: w766 -> [_ _ _ w816 _]
                              tunnel: w765 -> [_ _ _ w826 _]
                              tunnel: w764 -> [_ _ _ w825 _]
                              tunnel: w763 -> [_ _ _ _ _]
                              tunnel: w762 -> [_ _ _ _ w832]
                              frame #0 {
                                w775 = "\\"
                                n546 = case shown="\"CHART TEST\", Default" w788 {
                                tunnel: ["L01-1-CHART TEST-" "L01-1-CYCLE TEST-" "L01-1-T-RISE TEST-"] -> w784
                                frame "CHART TEST", Default {
                                }
                                frame "CYCLE TEST" {
                                }
                                frame "T-RISE TEST" {
                                }
                                }
                                n547 = local read "SET LAB01-1"() -> (w783:T5)
                                n548 = Unbundle(w783) -> ("DESCRIPTION"=w782:string)  [unwired: 4 out]
                                n549 = Concatenate Strings(w778, "\\", w776, w775, w774, w775) -> (w785:string)
                                n550 = String To Path(string=w785) -> (path=w787:path)
                                n551 = Concatenate Strings(w785, w784, w782, "-", w781, ".tdms") -> (w773:string)
                                n552 = Create Folder(path (use dialog)=w787) -> (error out=w786:errorcluster)  [unwired: 2 in, 2 out]
                                n553 = call <vilib>:"Clear Errors.vi"("error in (no error)"=w786) -> ()  [unwired: 6 in, 1 out]
                                n554 = global write "Global 1.vi" "LAB01-1 FILE"(w773) -> ()
                              }
                              frame #1 {
                                (unwired) FALSE
                                n555 = String To Path(string=w794) -> (path=w792:path)
                                n556 = TDMS Open(6:FALSE, 10:T21."create or replace" ("operation (0:open)"), 11:w792) -> (0:w795:errorcluster, 3:→"TDMS LAB01-1":refnum<k34>)  [unwired: 4 in]
                              }
                              frame #2 {
                                n557 = local read "TDMS LAB01-1"() -> (w814:refnum<k34>)
                                n558 = local read "SET LAB01-1"() -> (w803:T5)
                                n559 = Build Array("Testers Name", "Description", "Set Test Cycles", "T-Rise minutes", "T-Rise Deg C") -> (w804:string[])
                                n560 = Unbundle(w803) -> ("NAME"=w802:string, "DESCRIPTION"=w801:string, "CYCLES"=w800:dbl, "T-RISE mins"=w799:dbl, "T-RISE deg C"=w798:dbl)
                                n561 = Number To Decimal String(number=w800) -> (decimal integer string=w813:string)  [unwired: 1 in]
                                n562 = Number To Decimal String(number=w799) -> (decimal integer string=w812:string)  [unwired: 1 in]
                                n563 = Number To Decimal String(number=w798) -> (decimal integer string=w811:string)  [unwired: 1 in]
                                n564 = Build Array(w802, w801, w813, w812, w811) -> (w810:string[])
                                n565 = TDMS Set Properties(5:w810, 7:w804, 11:w814) -> ()  [unwired: 3 in, 4 out]
                              }
                              frame #3 {
                                n566 = local read "DISP LAB01-1"() -> (w824:T4)
                                n567 = Concatenate Strings("LAB01-1  ", w816) -> (w815:string)
                                n568 = Two Button Dialog(message=w815, 1:w825, 2:w826) -> (T button?=w818:bool)
                                n569 = case shown="True" w818 {
                                tunnel: w824 -> [w829 w830]
                                tunnel: [w829 w830] -> w823
                                tunnel: [w828 w831] -> w822
                                tunnel: [w827 w831] -> w821
                                frame False {
                                n570 = Unbundle(w829) -> ("CYCLE"=w828:dbl, "MINS"=w827:dbl)  [unwired: 1 out]
                                }
                                frame True {
                                w831 = 0.0
                                }
                                }
                                n571 = Bundle(cluster=w823, "CYCLE"=w822, "MINS"=w821, "STATUS"="RUN") -> (w820:T4)
                                n572 = local write "DISP LAB01-1"(w820) -> ()
                              }
                              frame #4 {
                                n573 = local read "TEMP START LAB01-1"() -> (w834:cluster{"TL":dbl, "TN":dbl})
                                n574 = Bundle(cluster=w834, "TL"=w832, "TN"=w832) -> (w833:cluster{"TL":dbl, "TN":dbl})
                                n575 = local write "TEMP START LAB01-1"(w833) -> ()
                              }
                            }
                          }
                        }
                      }
                    }
                  }
                }
              }
              event "RUN LAB01-2": Value Change {
                n576 = event-data() -> ("NewVal"=w839:bool)  [unwired: 1 in, 5 out]
                n577 = local write "run lab01-2"(w839) -> ()
                n578 = case shown="True" w839 {
